vi "set Parameter Licor Commands.vi"(0 "Licor-Commands":T4=enum."calibration-Z-H2O", 11 "command parameter":T1={"CO2 ref"=392.0, "CO2 span"=372.0, "H2O ref"=0.0, "H2O span"=0.0, "Zi"=0.0, "Zt"=1.2, "Zm"=0.0, "S"=0.0, "Temp [C]"=50.0, "Pressure [hPa]"=135.0, "Licor-Sources"=["CO2A W", "CO2B W", "H2OA W", "H2OB W", "T C", "T V", "P kPa", "P V", "RH %", "CO2A um/m", "CO2B um/m", "H2OA mm/m", "H2OB mm/m"], "Licor-Pump"="Off", "Zeitstempel"=timestamp(0 s since 1904-01-01)} {"Pressure [hPa]" format="%_5g"; "Temp [C]" format="%.2f"; "CO2 ref" format="%.2f"; "CO2 span" format="%.2g"; "H2O ref" format="%.2g"; "H2O span" format="%.2g"; "Zt" format="%#_4g"}) -> (4 "command":string)   [LabVIEW 2017, in "Licor-Steuerung.lvlib"]
uses:
  Licor-Steuerung.lvlib
  Licor-Commands.ctl
  Licor-Parameter.ctl
  LicorLI7000/conventions/Licor-Source.ctl
  Licor-Pump.ctl
  LicorLI7000/LicorLI7000.lvlib
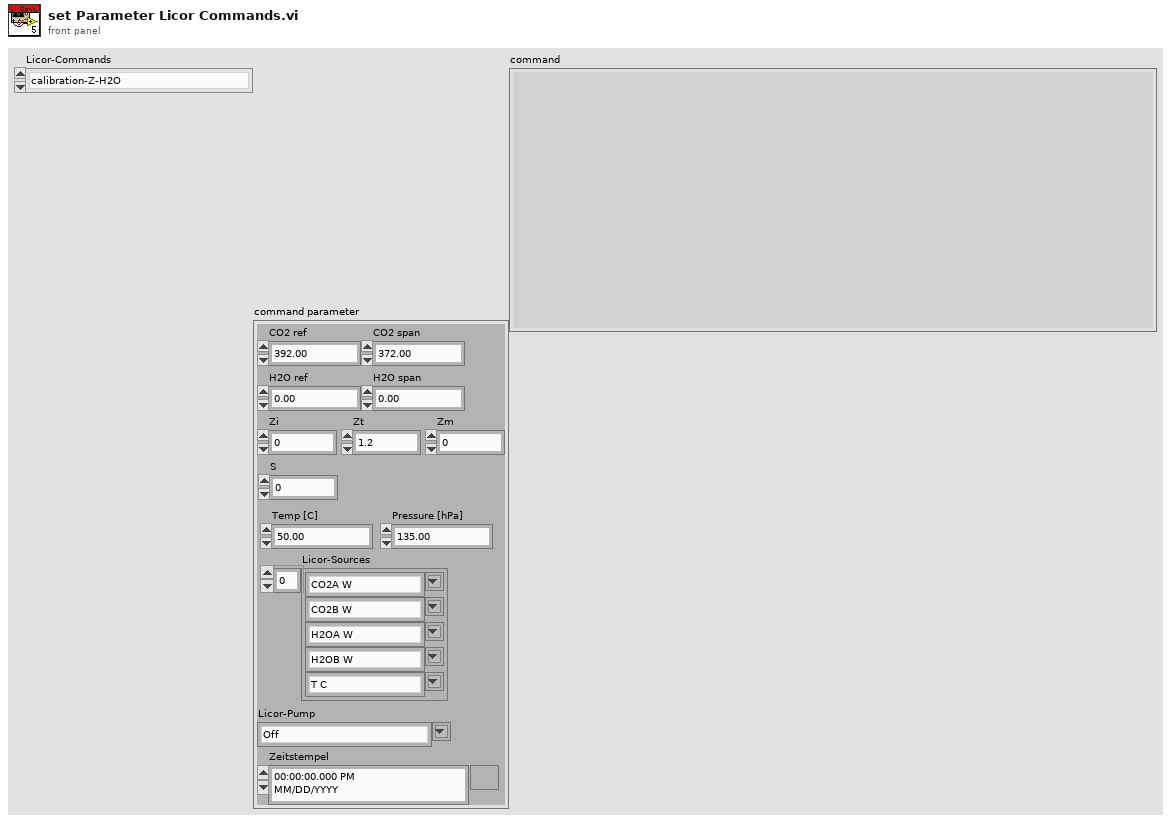
[diagram p1: front panel]
types:
  T1 = typedef "Licor-Steuerung.lvlib/Licor-Parameter.ctl" = cluster{"CO2 ref":dbl, "CO2 span":dbl, "H2O ref":dbl, "H2O span":dbl, "Zi":dbl, "Zt":dbl, "Zm":dbl, "S":dbl, "Temp [C]":dbl, "Pressure [hPa]":dbl, "Licor-Sources":T2[], "Licor-Pump":T3, "Zeitstempel":timestamp}
  T2 = typedef "LicorLI7000.lvlib/Licor-Source.ctl" = string
  T3 = typedef "Licor-Steuerung.lvlib/Licor-Pump.ctl" = string
  T4 = typedef "Licor-Steuerung.lvlib/Licor-Commands.ctl" = enum16{"wait", "initialize", "resetCO2", "resetH2O", "getReference", "setReference", "calibration-Z-CO2", "calibration-Z-H2O", "calibration-S-CO2", "calibration-S-H2O", "getCalibrationParameter", "setZeroParameter", "setLicorTime", "getLicorTime", "setPumpFlowrate", "setPumpSlow", "setPumpMedium", "setPumpFast", "getInfo"}
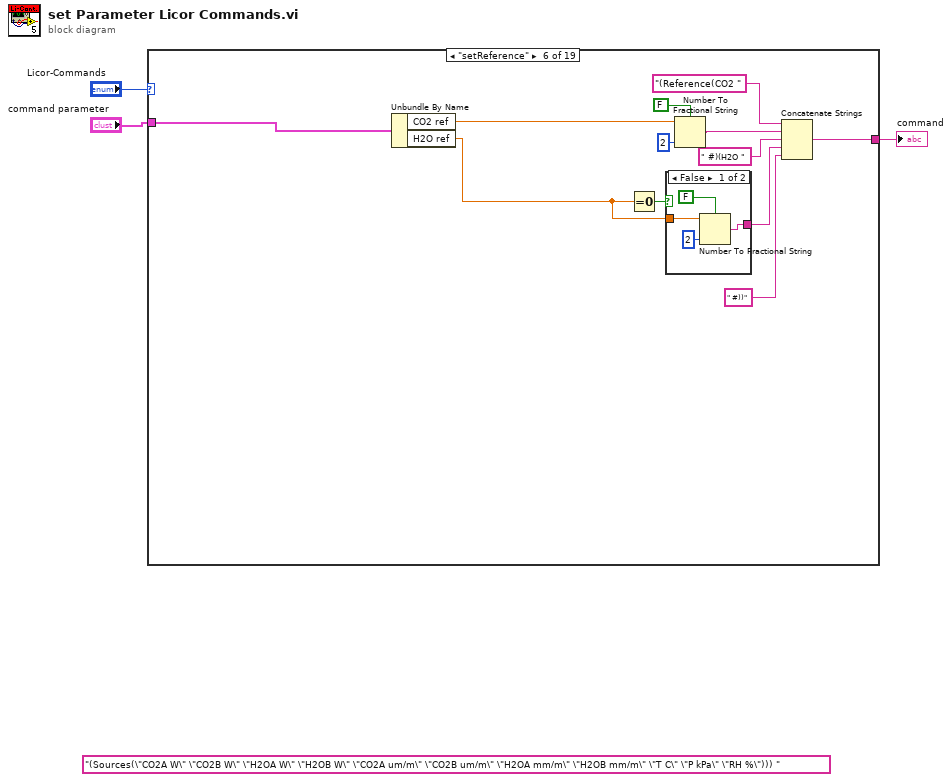
[diagram p0: block diagram]
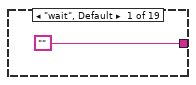
[diagram p2: hidden frame]
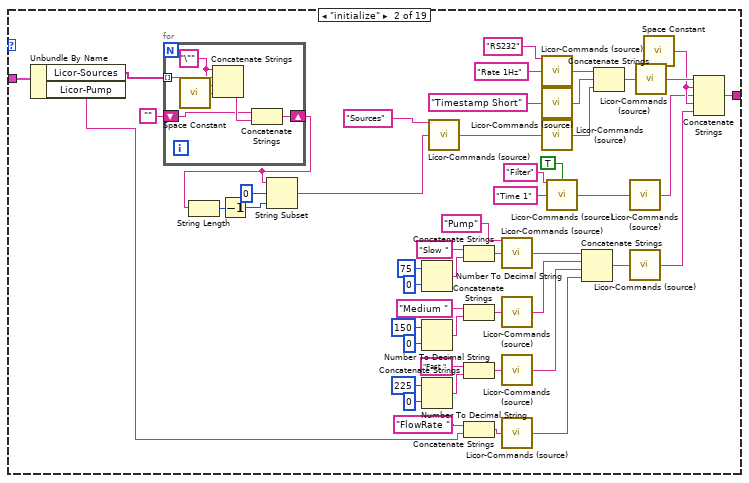
[diagram p3: hidden frame]
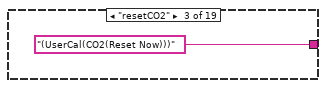
[diagram p4: hidden frame]
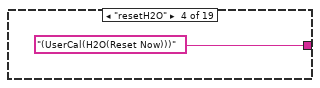
[diagram p5: hidden frame]
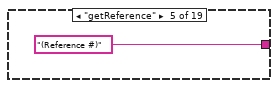
[diagram p6: hidden frame]
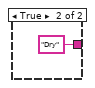
[diagram p7: hidden frame]
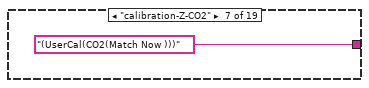
[diagram p8: hidden frame]
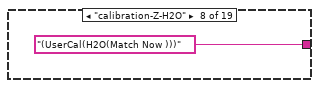
[diagram p9: hidden frame]
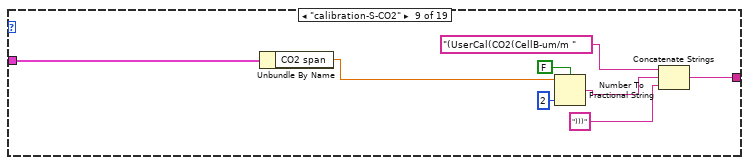
[diagram p10: hidden frame]
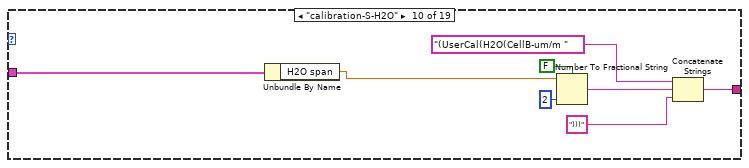
[diagram p11: hidden frame]
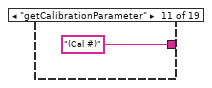
[diagram p12: hidden frame]
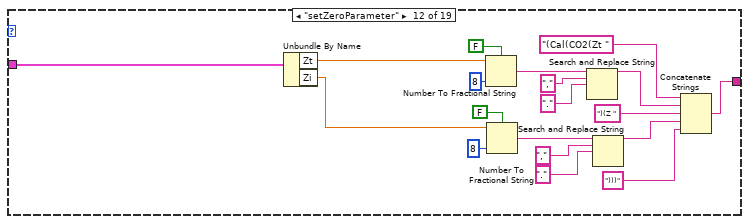
[diagram p13: hidden frame]
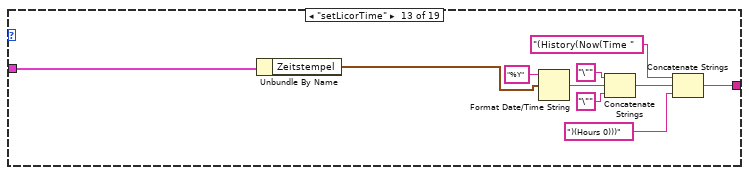
[diagram p14: hidden frame]
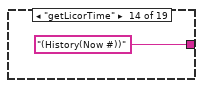
[diagram p15: hidden frame]
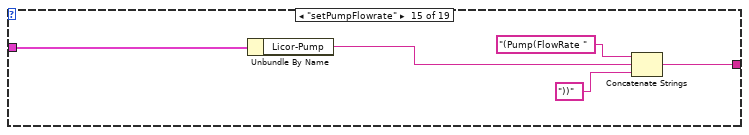
[diagram p16: hidden frame]
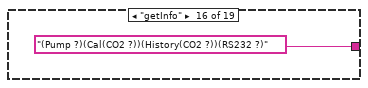
[diagram p17: hidden frame]
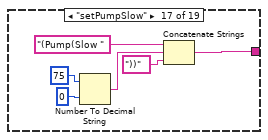
[diagram p18: hidden frame]
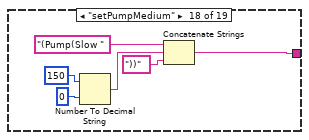
[diagram p19: hidden frame]
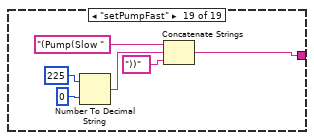
[diagram p20: hidden frame]
diagram:
  (unwired) "(Sources(\"CO2A W\" \"CO2B W\" \"H2OA W\" \"H2OB W\" \"CO2A um/m\" \"CO2B um/m\" \"H2OA mm/m\" \"H2OB mm/m\" \"T C\" \"P kPa\" \"RH %\"))) "
  n1 = case shown="\"setReference\"" "Licor-Commands" {
    tunnel: ["" w16 "(UserCal(CO2(Reset Now)))" "(UserCal(H2O(Reset Now)))" "(Reference #)" ("Befehl") w70 "(UserCal(CO2(Match Now )))" ("Befehl") "(UserCal(H2O(Match Now )))" ("Befehl") w88 w96 "(Cal #)" ("Befehl") w105 w128 "(History(Now #))" ("Befehl") w134 "(Pump ?)(Cal(CO2 ?))(History(CO2 ?))(RS232 ?)" ("Befehl") w136 w142 w148] -> w3
    tunnel: "command parameter" -> [_ w13 _ _ _ w69 _ _ w87 w95 _ w104 w120 _ w131 _ _ _ _]
    frame "wait", Default {
    }
    frame "initialize" {
      n2 = Unbundle By Name(w13) -> ("Licor-Sources"=w12:T2[], "Licor-Pump"=w5:T3)
      n3 = for {
        tunnel: w12 -> [w60] mode=indexing
        shift-right: [w56] -> w8
        shift-left: "" -> [w55]
        w59 = "\""
        n4 = call <vilib>:"Space Constant.vi"() -> ("String"=w58:string)
        n5 = Concatenate Strings(w59, w60, w59, w58) -> (w57:string)
        n6 = Concatenate Strings(w55, w57) -> (w56:string)
      }
      n7 = String Length(string=w8) -> (length=w10:i32)
      n8 = Decrement(x=w10) -> (x-1=w9:i32)
      n9 = String Subset(string=w8, offset (0)=0 ("Offset (0)"), length (rest)=w9) -> (substring=w6:string)
      n10 = Number To Decimal String(number=75 ("Wert"), width (-)=i16 0 ("Breite (-)")) -> (decimal integer string=w46:string)
      n11 = Number To Decimal String(number=150 ("Wert"), width (-)=i16 0 ("Breite (-)")) -> (decimal integer string=w41:string)
      n12 = Number To Decimal String(number=225 ("Wert"), width (-)=i16 0 ("Breite (-)")) -> (decimal integer string=w36:string)
      n13 = call "Licor-Commands (source).vi"("type"="Sources" ("Type"), "value"=w6) -> ("out"=w51:string)  [unwired: 13 in]
      n14 = Concatenate Strings("Slow " ("Befehl"), w46) -> (w45:string)
      n15 = Concatenate Strings("Medium " ("Befehl"), w41) -> (w40:string)
      n16 = Concatenate Strings("Fast " ("Befehl"), w36) -> (w35:string)
      n17 = Concatenate Strings("FlowRate " ("Befehl"), w5) -> (w33:string)
      n18 = call "Licor-Commands (source).vi"("type"="Pump" ("Type"), "value"=w45) -> ("out"=w32:string)  [unwired: 13 in]
      n19 = call "Licor-Commands (source).vi"("value"=w40) -> ("out"=w31:string)  [unwired: 14 in]
      n20 = call "Licor-Commands (source).vi"("value"=w35) -> ("out"=w30:string)  [unwired: 14 in]
      n21 = call "Licor-Commands (source).vi"("value"=w33) -> ("out"=w29:string)  [unwired: 14 in]
      n22 = call "Licor-Commands (source).vi"("type"="RS232", "value"="Rate 1Hz") -> ("out"=w50:string)  [unwired: 13 in]
      n23 = call "Licor-Commands (source).vi"("value"="Timestamp Short") -> ("out"=w27:string)  [unwired: 14 in]
      n24 = call "Licor-Commands (source).vi"("value"=w51) -> ("out"=w26:string)  [unwired: 14 in]
      n25 = call "Licor-Commands (source).vi"("type"="Filter", "response?"=TRUE, "value"="Time 1") -> ("out"=w19:string)  [unwired: 12 in]
      n26 = Concatenate Strings(w32, w31, w30, w29) -> (w28:string)
      n27 = Concatenate Strings(w50, w27, w26) -> (w24:string)
      n28 = call "Licor-Commands (source).vi"("value"=w19) -> ("out"=w18:string)  [unwired: 14 in]
      n29 = call "Licor-Commands (source).vi"("value"=w28) -> ("out"=w17:string)  [unwired: 14 in]
      n30 = call "Licor-Commands (source).vi"("value"=w24) -> ("out"=w23:string)  [unwired: 14 in]
      n31 = call <vilib>:"Space Constant.vi"() -> ("String"=w22:string)
      n32 = Concatenate Strings(w23, w22, w18, w22, w17) -> (w16:string)
    }
    frame "resetCO2" {
    }
    frame "resetH2O" {
    }
    frame "getReference" {
    }
    frame "setReference" {
      n33 = Unbundle By Name(w69) -> ("CO2 ref"=w67:dbl, "H2O ref"=w64:dbl)
      n34 = Equal To 0?(x=w64) -> (x = 0?=w72:bool)
      n35 = case shown="False" w72 {
        tunnel: [w77 "Dry"] -> w73
        tunnel: w64 -> [w78 _]
        frame False {
          n36 = Number To Fractional String(use system decimal point (T)=FALSE ("Systemdezimalzeichen verwenden (T)"), number=w78, precision (6)=i16 2 ("Genauigkeit (6)")) -> (F-format string=w77:string)  [unwired: 1 in]
        }
        frame True {
        }
      }
      n37 = Number To Fractional String(use system decimal point (T)=FALSE ("Systemdezimalzeichen verwenden (T)"), number=w67, precision (6)=i16 2 ("Genauigkeit (6)")) -> (F-format string=w66:string)  [unwired: 1 in]
      n38 = Concatenate Strings("(Reference(CO2 " ("String"), w66, " #)(H2O " ("String"), w73, " #))" ("String")) -> (w70:string)
    }
    frame "calibration-Z-CO2" {
    }
    frame "calibration-Z-H2O" {
    }
    frame "calibration-S-CO2" {
      n39 = Unbundle By Name(w87) -> ("CO2 span"=w83:dbl)
      n40 = Number To Fractional String(use system decimal point (T)=FALSE ("Systemdezimalzeichen verwenden (T)"), number=w83, precision (6)=i16 2 ("Genauigkeit (6)")) -> (F-format string=w84:string)  [unwired: 1 in]
      n41 = Concatenate Strings("(UserCal(CO2(CellB-um/m " ("Befehl"), w84, ")))" ("Befehl")) -> (w88:string)
    }
    frame "calibration-S-H2O" {
      n42 = Unbundle By Name(w95) -> ("H2O span"=w91:dbl)
      n43 = Number To Fractional String(use system decimal point (T)=FALSE ("Systemdezimalzeichen verwenden (T)"), number=w91, precision (6)=i16 2 ("Genauigkeit (6)")) -> (F-format string=w92:string)  [unwired: 1 in]
      n44 = Concatenate Strings("(UserCal(H2O(CellB-um/m " ("Befehl"), w92, ")))" ("Befehl")) -> (w96:string)
    }
    frame "getCalibrationParameter" {
    }
    frame "setZeroParameter" {
      n45 = Unbundle By Name(w104) -> ("Zt"=w103:dbl, "Zi"=w100:dbl)
      n46 = Number To Fractional String(use system decimal point (T)=FALSE ("Systemdezimalzeichen verwenden (T)"), number=w103, precision (6)=i16 8 ("Genauigkeit (6)")) -> (F-format string=w115:string)  [unwired: 1 in]
      n47 = Number To Fractional String(use system decimal point (T)=FALSE ("Systemdezimalzeichen verwenden (T)"), number=w100, precision (6)=i16 8 ("Genauigkeit (6)")) -> (F-format string=w108:string)  [unwired: 1 in]
      n48 = Search and Replace String(input string=w115, search string="," ("Such-String"), replace string="." ("Ersetzungs-String (\"\")")) -> (result string=w114:string)  [unwired: 5 in, 3 out]
      n49 = Search and Replace String(input string=w108, search string="," ("Such-String"), replace string="." ("Ersetzungs-String (\"\")")) -> (result string=w107:string)  [unwired: 5 in, 3 out]
      n50 = Concatenate Strings("(Cal(CO2(Zt " ("Befehl"), w114, ")(Z " ("Befehl"), w107, ")))" ("Befehl")) -> (w105:string)
    }
    frame "setLicorTime" {
      n51 = Unbundle By Name(w120) -> ("Zeitstempel"=w119:timestamp)
      n52 = Format Date/Time String(time format string (%c)="%Y" ("Zeitformatierungs-String (%c)"), seconds (now)=w119) -> (date/time string=w125:string)  [unwired: 1 in]
      n53 = Concatenate Strings("\"" ("String"), w125, "\"" ("String")) -> (w122:string)
      n54 = Concatenate Strings("(History(Now(Time " ("Befehl"), w122, ")(Hours 0)))" ("Befehl")) -> (w128:string)
    }
    frame "getLicorTime" {
    }
    frame "setPumpFlowrate" {
      n55 = Unbundle By Name(w131) -> ("Licor-Pump"=w130:T3)
      n56 = Concatenate Strings("(Pump(FlowRate " ("Befehl"), w130, "))" ("Befehl")) -> (w134:string)
    }
    frame "getInfo" {
    }
    frame "setPumpSlow" {
      n57 = Number To Decimal String(number=75 ("Wert"), width (-)=i16 0 ("Breite (-)")) -> (decimal integer string=w137:string)
      n58 = Concatenate Strings("(Pump(Slow " ("Befehl"), w137, "))" ("Befehl")) -> (w136:string)
    }
    frame "setPumpMedium" {
      n59 = Number To Decimal String(number=150 ("Wert"), width (-)=i16 0 ("Breite (-)")) -> (decimal integer string=w143:string)
      n60 = Concatenate Strings("(Pump(Slow " ("Befehl"), w143, "))" ("Befehl")) -> (w142:string)
    }
    frame "setPumpFast" {
      n61 = Number To Decimal String(number=225 ("Wert"), width (-)=i16 0 ("Breite (-)")) -> (decimal integer string=w149:string)
      n62 = Concatenate Strings("(Pump(Slow " ("Befehl"), w149, "))" ("Befehl")) -> (w148:string)
    }
  }
  "command" <- w3
